vi "pythone code run for live scar detection.vi"(8 "error in (no error)":errorcluster) -> (0 "error out":errorcluster)   [LabVIEW 2025]
panel:
  out "return value":string
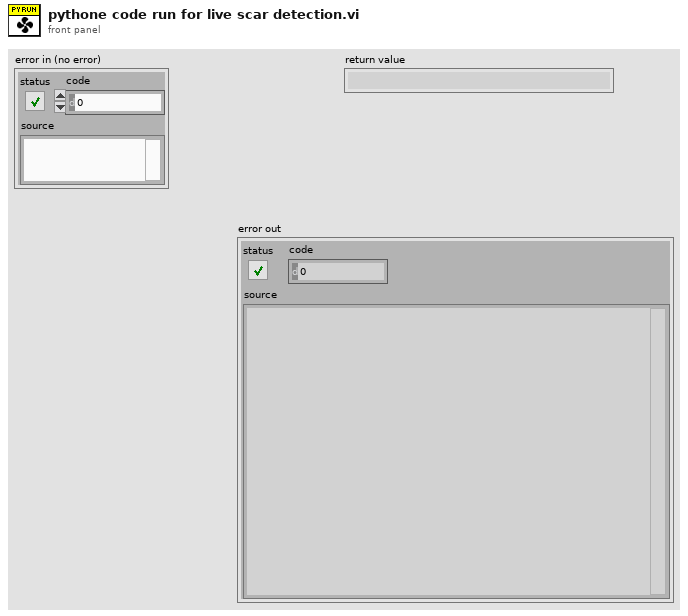
[diagram p1: front panel]
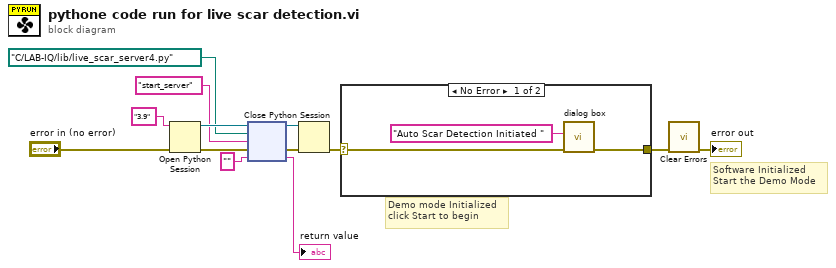
[diagram p0: block diagram]
diagram:
  # "Software Initialized\nStart the Demo Mode"
  # "Demo mode Initialized\nclick Start to begin"
  n1 = Open Python Session(python version="3.9" ("Python version"), 3:"error in (no error)") -> (session out=w12:refnum<k35>, error out=w10:errorcluster)  [unwired: 1 in]
  n2 = node(w12, path "C:/LAB-IQ/lib/live_scar_server4.py" ("Python path"), "start_server" ("function name"), w10, "" ("function name")) -> (w8:refnum<k35>, w9:errorcluster, →"return value":string)  [unwired: 2 out]
  n3 = Close Python Session(session in=w8, error in=w9) -> (11:w2:errorcluster)
  n4 = case shown="No Error" w2 {
    selector: w2 -> [w16 _]
    tunnel: [w15 _] -> w1
    frame No Error {
      n5 = call "dialog box.vi"("Status"="Auto Scar Detection Initiated " ("message"), "error in"=w16) -> ("error out"=w15:errorcluster)  [unwired: 8 in]
    }
    frame Error {
    }
  }
  n6 = call <vilib>:"Clear Errors.vi"("error in (no error)"=w1) -> ("error out"=→"error out":errorcluster)  [unwired: 5 in, 1 out]
